vi "Color Detection.vi"() -> ()   [LabVIEW 2019]
uses:
  <vilib>/userDefined/High Color/IMAQdx.ctl
  <vilib>/vision/driver/NI_Vision_Acquisition_Software.lvlib
  <vilib>/vision/NI_Vision_Development_Module.lvlib
panel:
  out "YELLOW":bool
  out "BLACK":bool
  out "RED":bool
  out "BLUE":bool
  out "GREEN":bool
  out "Color Spectrum 2":dbl[](array[numeric]) format="%.2f"
  in  "stop":bool
  in  "Color Sensitivity":u32(ring) items=["Low", "Medium", "High"]
  out "Image":T1(plugin-control)
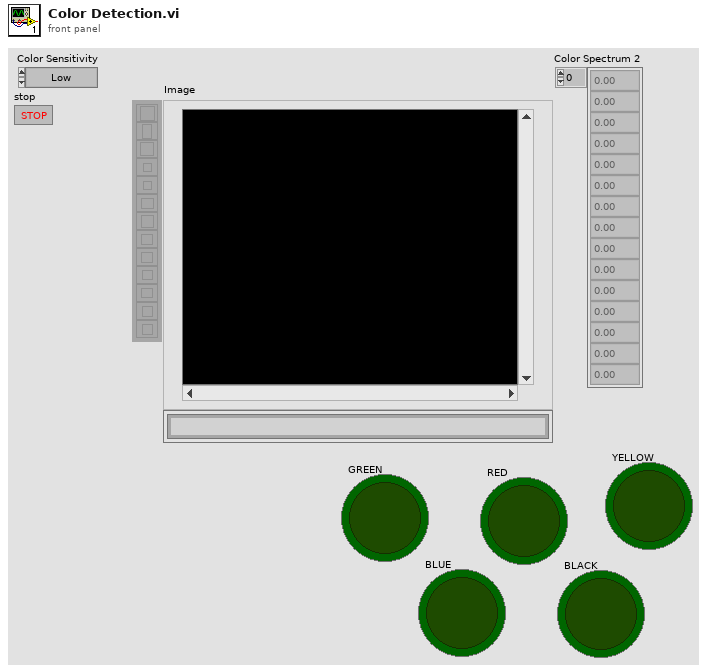
[diagram p1: front panel]
types:
  T1 = typedef "IMAQ Image.ctl" = refnum<image>
  T2 = typedef "IMAQdx.ctl" = refnum<k21>
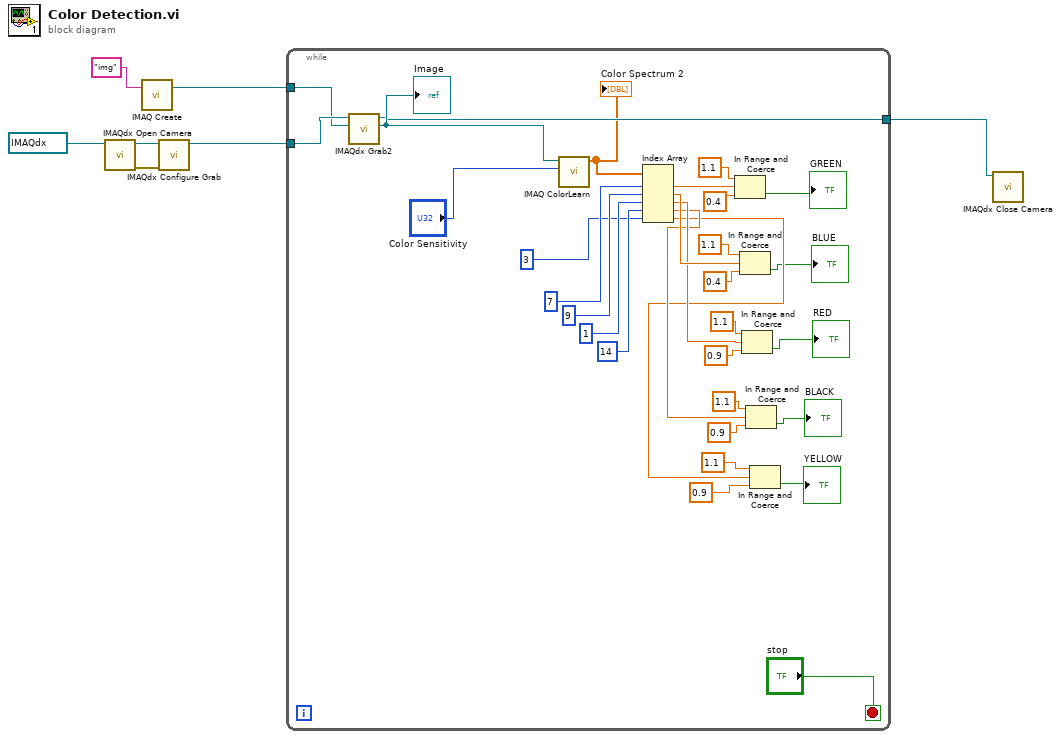
[diagram p0: block diagram]
diagram:
  n1 = call <vilib>:"IMAQdx Open Camera.vi"("Session In"=T2 "cam0") -> ("error out"=w4:errorcluster, "Session Out"=w3:T2)  [unwired: 9 in]
  n2 = call "IMAQ Create"("Image Name"="img") -> ("New Image"=w5:T1)  [unwired: 4 in, 1 out]
  n3 = call <vilib>:"IMAQdx Configure Grab.vi"("error in"=w4, "Session In"=w3) -> ("Session Out"=w2:T2)  [unwired: 8 in, 1 out]
  n4 = while {
    tunnel: w5 -> [w38]
    tunnel: w2 -> [w39]
    tunnel: [w35] -> w1
    stop <- "stop" stop-if-true
    n5 = call <vilib>:"IMAQdx Grab2.vi"("Image In"=w38, "Session In"=w39) -> ("Image Out"=w36:T1, "Session Out"=w35:T2)  [unwired: 6 in, 2 out]
    "Image" <- w36
    n6 = call "IMAQ ColorLearn"("Image"=w36, "Color Sensitivity"="Color Sensitivity") -> ("Color Spectrum"=w28:dbl[])  [unwired: 6 in, 1 out]
    "Color Spectrum 2" <- w28
    n7 = Index Array(array=w28, index #1=7 ("index"), index #2=9 ("index"), index #3=1 ("index"), index #4=14 ("index"), index #5=3 ("index")) -> (element #1=w27:dbl, element #2=w24:dbl, element #3=w21:dbl, element #4=w18:dbl, element #5=w15:dbl)
    n8 = In Range and Coerce(upper limit=1.1, x=w27, lower limit=0.4) -> (In Range?=→"GREEN":bool)  [unwired: 1 out]
    n9 = In Range and Coerce(upper limit=1.1, x=w24, lower limit=0.4) -> (In Range?=→"BLUE":bool)  [unwired: 1 out]
    n10 = In Range and Coerce(upper limit=1.1, x=w21, lower limit=0.9) -> (In Range?=→"RED":bool)  [unwired: 1 out]
    n11 = In Range and Coerce(upper limit=1.1, x=w18, lower limit=0.9) -> (In Range?=→"BLACK":bool)  [unwired: 1 out]
    n12 = In Range and Coerce(upper limit=1.1, x=w15, lower limit=0.9) -> (In Range?=→"YELLOW":bool)  [unwired: 1 out]
  }
  n13 = call <vilib>:"IMAQdx Close Camera.vi"("Session In"=w1) -> ()  [unwired: 10 in, 1 out]
